vi "Tthermistor Vdc.vi"(5 "ThermConfig":T1, 7 "thermCirc":T2={"Vsource"=10.0, "SH Coeff"=[0.0010291947674223878, 0.00023912751839781632, 1.5662771497033316e-07], "R1"=10.0, "Rref"=[], "Tref"=[]}, 8 "Init":bool=TRUE, 9 "Vdc":dbl[](array[numeric])=[2.4400000000000004]) -> (2 "Rt":dbl[](array[numeric])=[38770.49180327869], 3 "T":dbl[](array[numeric])=[-5.7990766588590645])   [LabVIEW 2015, in "Temperature.lvlib"]
doc: "Converts the voltage measured off of a thermistor circuit consisting of a voltage divider using the the Steinhart-Hart coefficients for the appropriate thermistor."
uses:
  Temperature.lvlib
  Thermistor Config.ctl
  Thermistor Position.ctl
  Convert V to Rt - DBL Array.vi
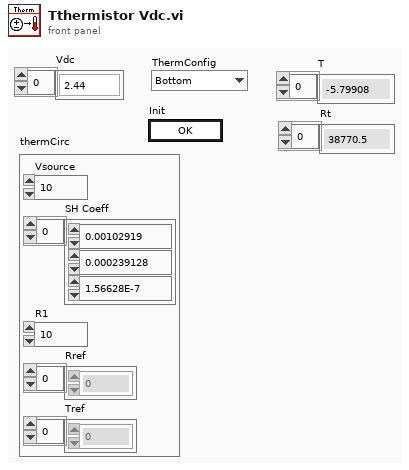
[diagram p1: front panel]
types:
  T1 = typedef "Temperature.lvlib/Thermistor Position.ctl" = enum8{"Bottom", "Top"}
  T2 = typedef "Temperature.lvlib/Thermistor Config.ctl" = cluster{"Vsource":dbl, "SH Coeff":dbl[], "R1":dbl, "Rref":dbl[], "Tref":dbl[]}
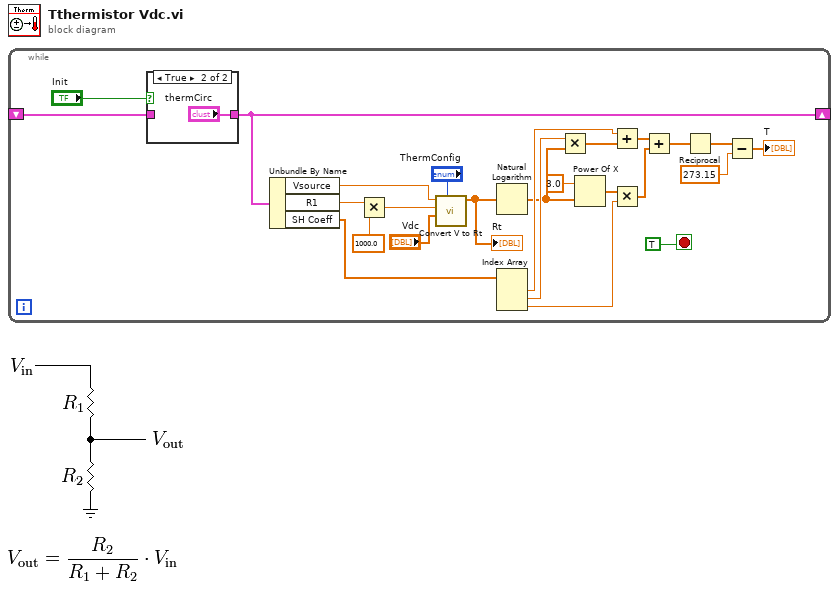
[diagram p0: block diagram]
diagram:
  n1 = while {
    shift-right: [w10] -> _
    shift-left: _ -> [w11]
    stop <- TRUE stop-if-true
    n2 = case shown="True" "Init" {
      tunnel: w11 -> [w26 _]
      tunnel: [w26 "thermCirc"] -> w10
      frame False {
      }
      frame True {
      }
    }
    n3 = Unbundle By Name(w10) -> ("Vsource"=w2:dbl, "R1"=w4:dbl, "SH Coeff"=w9:dbl[])
    n4 = Multiply(x=w4, y=1000.0 ("Convert to Ohms")) -> (x*y=w7:dbl)
    n5 = call-poly "Convert V to Rt.vi"("ThermConfig"="ThermConfig", "Vmeas"="Vdc", "Rref"=w7, "Vsource"=w2) -> ("Rt"=w6:dbl[])  [unwired: 7 in]
    "Rt" <- w6
    n6 = Natural Logarithm(1:w6) -> (0:w20:dbl[])
    n7 = Index Array(array=w9) -> (element #1=w23:dbl, element #2=w22:dbl, element #3=w17:dbl)  [unwired: 3 in]
    n8 = Multiply(x=w22, y=w20) -> (x*y=w16:dbl[])
    n9 = Power Of X(1:w20, 2:3.0 ("y")) -> (0:w18:dbl[])
    n10 = Add(x=w23, y=w16) -> (x+y=w19:dbl[])
    n11 = Multiply(x=w18, y=w17) -> (x*y=w15:dbl[])
    n12 = Add(x=w19, y=w15) -> (x+y=w14:dbl[])
    n13 = Reciprocal(x=w14) -> (1/x=w25:dbl[])
    n14 = Subtract(x=w25, y=273.15) -> (x-y=→"T":dbl[])
  }
